vi "Enable Controls.vi"(8 "error in (no error)":errorcluster, 11 "Enable Disable":T1(ring)) -> (0 "error out":errorcluster)   [LabVIEW 2020]
doc: "Author: Scott Hannahs <sth@magnet.fsu.edu>\nCopyright 2018 Florida State University, All rights reserved."
uses:
  Interlock 32T Net Client Globals.vi
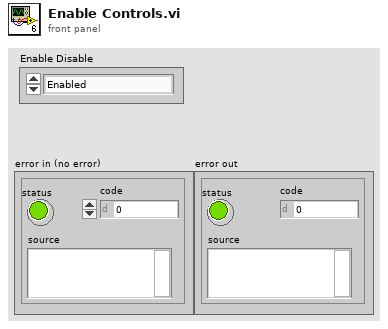
[diagram p1: front panel]
types:
  T1 = enum8{"Enabled", "Disabled", "Disabled and Grayed Out"}
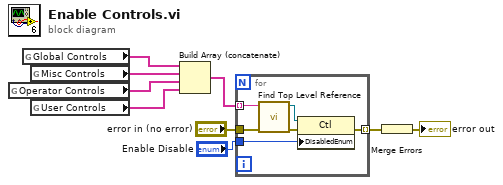
[diagram p0: block diagram]
diagram:
  n1 = global read "Interlock 32T Net Client Globals.vi" "Operator Controls"() -> (w2:string[])
  n2 = global read "Interlock 32T Net Client Globals.vi" "Global Controls"() -> (w8:string[])
  n3 = global read "Interlock 32T Net Client Globals.vi" "Misc Controls"() -> (w3:string[])
  n4 = global read "Interlock 32T Net Client Globals.vi" "User Controls"() -> (w1:string[])
  n5 = Build Array (concatenate)(w8, w3, w2, w1) -> (w9:string[])
  n6 = for {
    tunnel: "Enable Disable" -> [w14]
    tunnel: w9 -> [w12] mode=indexing
    tunnel: [w11] -> w5 mode=indexing
    tunnel: "error in (no error)" -> [w10]
    n7 = call "Find Top Level Reference.vi"("error in (no error)"=w10, "String"=w12) -> ("error out"=w13:errorcluster, "Ctl Refnum"=w15:refnum<vi>)  [unwired: 8 in]
    n8 = property on="Property Node" class="Ctl"(reference=w15, error in=w13, "DisabledEnum"=w14) -> (error out=w11:errorcluster)  [unwired: 1 out]
  }
  n9 = Merge Errors(w5) -> (→"error out":errorcluster)
